vi "MessengerBecameInvalid Event.vi"(10 "MGR became Invalid":refnum<user-event>, 11 "Messenger":refnum<class "MGR.lvclass">) -> ()   [LabVIEW 2011, in "Messenging.lvlib" / "Parallel Process.lvclass"]
uses:
  Parallel Process.lvclass
  Interprocess Messenger/Messenger (Parent)/MGR.lvclass
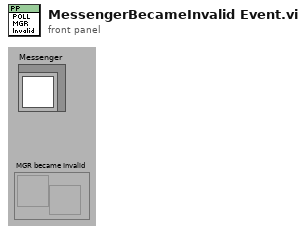
[diagram p1: front panel]
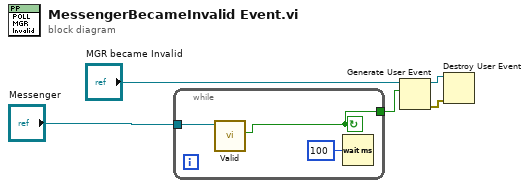
[diagram p0: block diagram]
diagram:
  n1 = while {
    tunnel: "Messenger" -> [w7]
    tunnel: [w6] -> w4
    stop <- w6 continue-if-true
    n2 = call-dynamic "Valid.vi"("Send in"=w7) -> ("Valid?"=w6:bool)  [unwired: 10 out]
    n3 = Wait (ms)(milliseconds to wait=u32 100) -> ()  [unwired: 1 out]
  }
  n4 = Generate User Event(user event="MGR became Invalid", event data cluster=w4) -> (user event out=w1:refnum<user-event>, error out=w2:errorcluster)  [unwired: 1 in]
  n5 = Destroy User Event(user event=w1, error in=w2) -> ()  [unwired: 1 out]
